vi "285A_GetPos.vi"(8 "error in (no error)":errorcluster caption="错误输入（无错误）", 11 "VISA资源名称":refnum<visa-resource-name>) -> (0 "error out":errorcluster caption="错误输出", 1 "Z":dbl, 2 "Y":dbl, 3 "X":dbl, 4 "read buffer":string, 5 "VISA资源名称输出":refnum<visa-resource-name>)   [LabVIEW 2016]
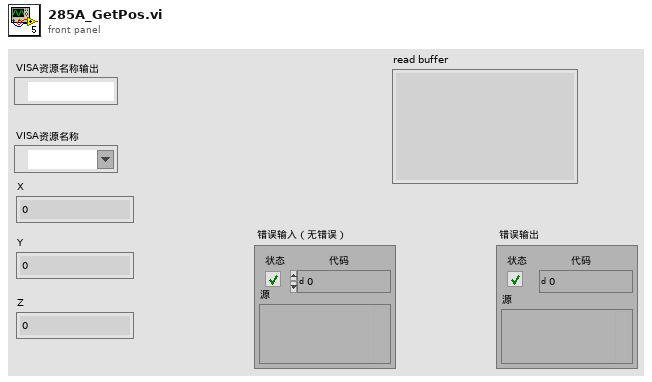
[diagram p1: front panel]
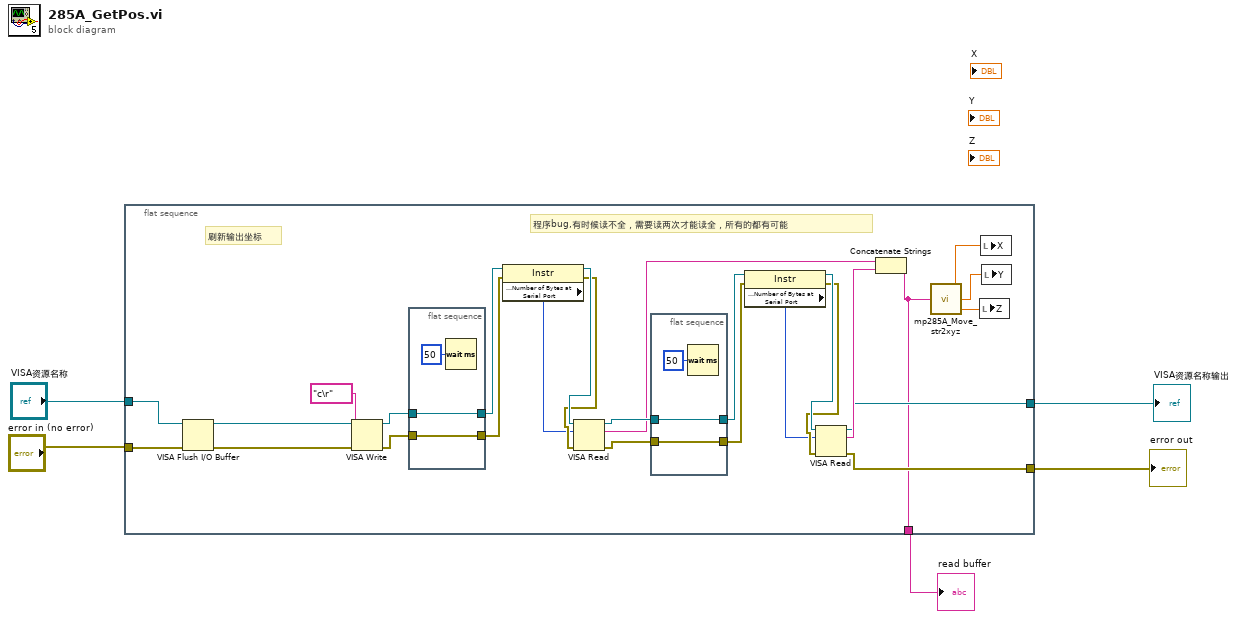
[diagram p0: block diagram]
diagram:
  n1 = flat-sequence {
    tunnel: "error in (no error)" -> [w26]
    tunnel: "VISA资源名称" -> [w27]
    tunnel: [w11] -> w3
    tunnel: [w10] -> w2
    tunnel: [w7] -> w1
    frame #0 {
      # "程序bug,有时候读不全，需要读两次才能读全，所有的都有可能"
      # "刷新输出坐标"
      n2 = VISA Flush I/O Buffer(VISA resource name=w27, error in (no error)=w26) -> (VISA resource name out=w29:refnum<visa-resource-name>, error out=w28:errorcluster)  [unwired: 1 in]
      n3 = VISA Write ("VISA写入")(VISA resource name=w29, write buffer="c\r" ("写入缓冲区"), error in (no error)=w28) -> (VISA resource name out=w31:refnum<visa-resource-name>, error out=w32:errorcluster)  [unwired: 1 out]
      n4 = flat-sequence {
        tunnel: [w37] -> w25
        tunnel: w31 -> [w37]
        tunnel: [w36] -> w24
        tunnel: w32 -> [w36]
        frame #0 {
          n5 = Wait (ms)(milliseconds to wait=u32 50 ("等待时间（毫秒）")) -> ()  [unwired: 1 out]
        }
      }
      n6 = property class="Instr"(reference=w25, error in=w24) -> (reference out=w23:refnum<visa-resource-name>, error out=w22:errorcluster, "Serial Settings:Number of Bytes at Serial Port"=w21:u32)
      n7 = VISA Read(VISA resource name=w23, byte count=w21, error in (no error)=w22) -> (VISA resource name out=w15:refnum<visa-resource-name>, read buffer=w13:string, error out=w14:errorcluster)  [unwired: 1 out]
      n8 = flat-sequence {
        tunnel: [w34] -> w20
        tunnel: w15 -> [w34]
        tunnel: [w33] -> w19
        tunnel: w14 -> [w33]
        frame #0 {
          n9 = Wait (ms)(milliseconds to wait=u32 50 ("等待时间（毫秒）")) -> ()  [unwired: 1 out]
        }
      }
      n10 = property class="Instr"(reference=w20, error in=w19) -> (reference out=w18:refnum<visa-resource-name>, error out=w17:errorcluster, "Serial Settings:Number of Bytes at Serial Port"=w16:u32)
      n11 = VISA Read(VISA resource name=w18, byte count=w16, error in (no error)=w17) -> (VISA resource name out=w11:refnum<visa-resource-name>, read buffer=w12:string, error out=w10:errorcluster)  [unwired: 1 out]
      n12 = Concatenate Strings(w13, w12) -> (w7:string)
      n13 = call "mp285A_Move_str2xyz.vi"("字符串"=w7) -> ("X轴"=w9:dbl, "Y轴"=w8:dbl, "Z轴"=w6:dbl)
      n14 = local write "Z"(w6) -> ()
      n15 = local write "X"(w9) -> ()
      n16 = local write "Y"(w8) -> ()
    }
  }
  "error out" <- w2
  "VISA资源名称输出" <- w3
  "read buffer" <- w1
